vi "MKS670_1000_main.vi"(7 "stop_external":refnum<vi>, 8 "input cluster":T1) -> ()   [LabVIEW 2019]
uses:
  cluster_ref_MKS670.ctl
panel:
  out "Alarm Status":u32(colorbox)
  in  "HI":dbl=500.0 format="%.1f"
  in  "HIHI":dbl=700.0 format="%.1f"
  in  "SMS":bool=TRUE
  out "status_log":bool caption="Status"
  in  "Logging":bool=TRUE
  in  "Meas. Interval":u32=1000 caption="ms"
  out "P Chart":waveform(dbl)[](graph)
  out "Last Updated":timestamp format="%<%Y-%m-%d %H:%M:%S>T"
  in  "VISA":refnum<visa-resource-name>="COM16"
  out "Status":bool
  in  "stop":bool
  out "Pressure":dbl caption="Torr"
  # "MKS 670 for MKS 690 / 1000 Torr"
  # "Torr"
  # "Torr"
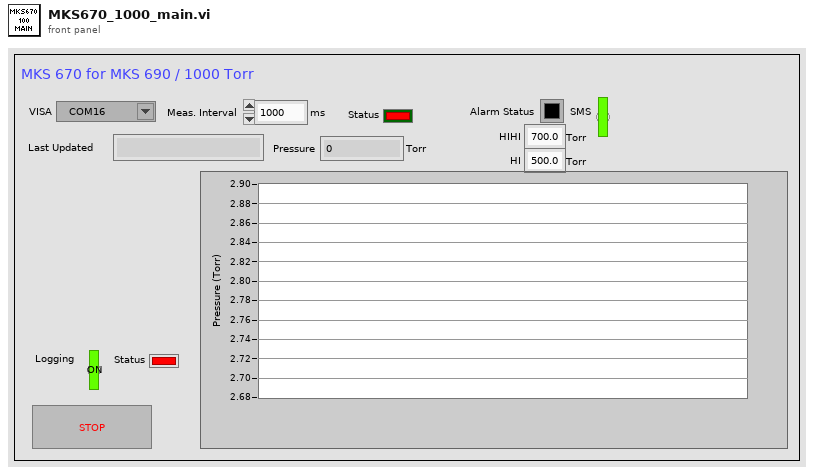
[diagram p1: front panel]
types:
  T1 = typedef "cluster_ref_MKS670.ctl" = cluster{"status":refnum<vi>, "PR":refnum<vi>}
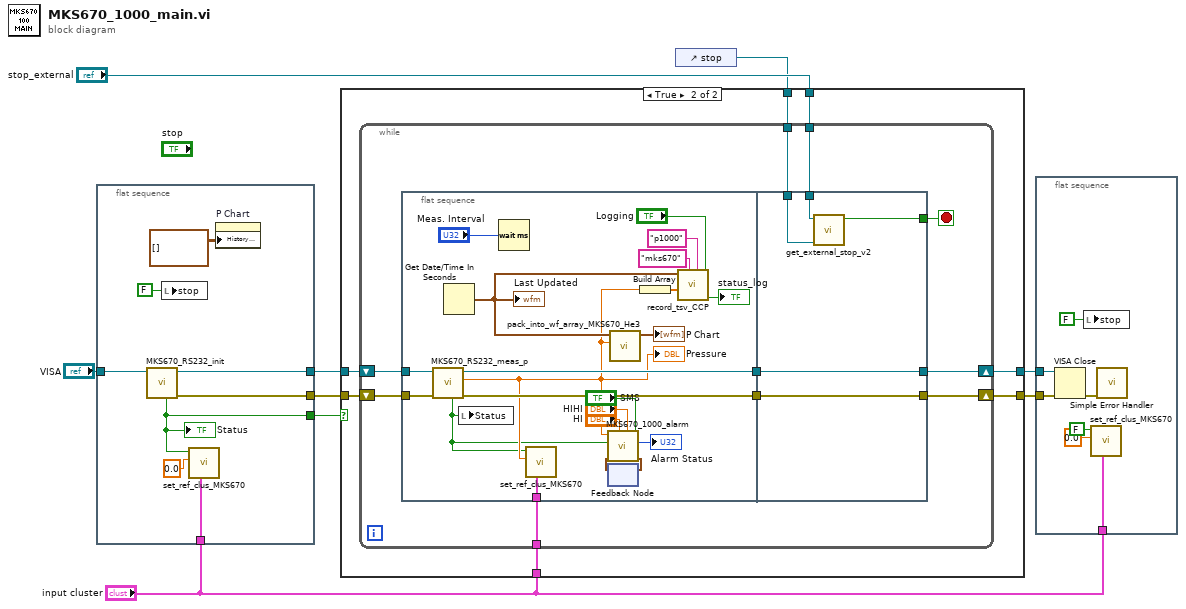
[diagram p0: block diagram]
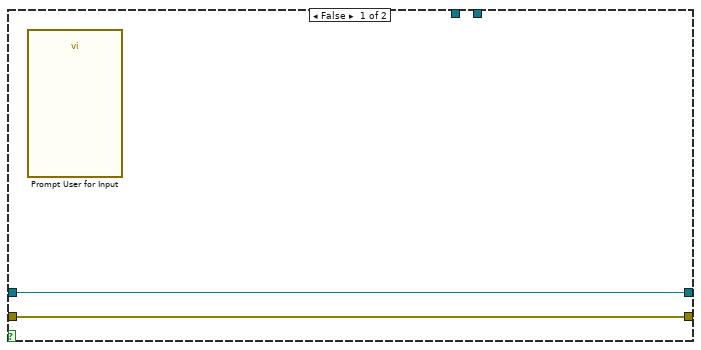
[diagram p2: hidden frame]
diagram:
  n1 = flat-sequence {
    tunnel: [w17] -> w9
    tunnel: "VISA" -> [w16]
    tunnel: [w15] -> w6
    tunnel: "input cluster" -> [w14]
    tunnel: [w12] -> w5
    frame #0 {
      n2 = call "MKS670_RS232_init.vi"("VISA in"=w16) -> ("error out"=w15:errorcluster, "VISA out"=w17:refnum<visa-resource-name>, "status"=w12:bool)  [unwired: 8 in]
      "Status" <- w12
      n3 = local write "stop"(FALSE ("stop")) -> ()
      n4 = call "set_ref_clus_MKS670.vi"("input cluster"=w14, "pressure"=0.0, "status"=w12) -> ()  [unwired: 9 in]
      n5 = property on="P Chart" class="WFChart (strict)"("History Data"=waveform(dbl)[][] []) -> ()  [unwired: 2 in, 2 out]
    }
  }
  n6 = control-ref of="stop"() -> (w2:refnum<vi>)
  n7 = case shown="True" w5 {
    tunnel: w9 -> [w19 w26]
    tunnel: "stop_external" -> [_ w25]
    tunnel: w6 -> [w18 w24]
    tunnel: "input cluster" -> [_ w23]
    tunnel: [w19 w22] -> w4
    tunnel: [w18 w21] -> w3
    tunnel: w2 -> [_ w20]
    frame False {
      n8 = call "Prompt User for Input"() -> ()  [unwired: 18 in, 2 out]
    }
    frame True {
      n9 = while {
        tunnel: w25 -> [w29]
        shift-right: [w34] -> w22
        shift-left: w26 -> [w36]
        shift-right: [w33] -> w21
        shift-left: w24 -> [w35]
        tunnel: w23 -> [w32]
        tunnel: w20 -> [w27]
        stop <- w28 stop-if-true
        n10 = flat-sequence {
          tunnel: w36 -> [w57]
          tunnel: w35 -> [w56]
          tunnel: w32 -> [w52]
          tunnel: [w55] -> w31
          tunnel: [w54] -> w30
          tunnel: [w61] -> w33
          tunnel: [w62] -> w34
          tunnel: w31 -> [w62]
          tunnel: w30 -> [w61]
          tunnel: w29 -> [w60]
          tunnel: [w59] -> w28
          tunnel: w27 -> [w58]
          frame #0 {
            n11 = call "MKS670_RS232_meas_p.vi"("error in"=w56, "VISA in"=w57) -> ("error out"=w54:errorcluster, "pressure"=w42:dbl, "VISA out"=w55:refnum<visa-resource-name>, "status"=w40:bool)  [unwired: 6 in]
            "Pressure" <- w42
            n12 = Get Date/Time In Seconds() -> (seconds since 1Jan1904=w50:timestamp)
            "Last Updated" <- w50
            n13 = local write "Status"(w40) -> ()
            n14 = Wait (ms)(milliseconds to wait="Meas. Interval") -> ()  [unwired: 1 out]
            n15 = call "set_ref_clus_MKS670.vi"("input cluster"=w52, "pressure"=w42, "status"=w40) -> ()  [unwired: 9 in]
            n16 = feedback #1() -> (w43:timestamp)  [unwired: 1 in]
            n17 = call "MKS670_1000_alarm.vi"("enabled"="SMS", "HIHI"="HIHI", "HI"="HI", "time_last_alarm_in"=w43, "readout_status"=w40, "P"=w42) -> ("time_last_alarm_out"=w44:timestamp, "alarm_status"=→"Alarm Status":u32)  [unwired: 4 in]
            n18 = feedback-in #1(w44) -> ()
            n19 = call "pack_into_wf_array_MKS670_He3.vi"("pressure"=w42, "time"=w50) -> ("waveform_array"=→"P Chart":waveform(dbl)[])  [unwired: 9 in]
            n20 = Build Array(w42) -> (w45:dbl[])
            n21 = call "record_tsv_CCP.vi"("logging_on"="Logging", "file_name"="p1000", "folder_name"="mks670", "value_array"=w45, "time"=w50) -> ("status"=→"status_log":bool)  [unwired: 5 in, 1 out]
          }
          frame #1 {
            n22 = call "get_external_stop_v2.vi"("ref_stop_internal"=w58, "ref_stop_external"=w60) -> ("stop_output"=w59:bool)  [unwired: 9 in]
          }
        }
      }
    }
  }
  n23 = flat-sequence {
    tunnel: w4 -> [w69]
    tunnel: w3 -> [w68]
    tunnel: "input cluster" -> [w66]
    frame #0 {
      n24 = VISA Close(VISA resource name=w69, error in (no error)=w68) -> (error out=w67:errorcluster)
      n25 = local write "stop"(FALSE ("stop")) -> ()
      n26 = call "set_ref_clus_MKS670.vi"("input cluster"=w66, "pressure"=0.0, "status"=FALSE) -> ()  [unwired: 9 in]
      n27 = call <vilib>:"Simple Error Handler.vi"("error in (no error)"=w67) -> ()  [unwired: 4 in, 5 out]
    }
  }
